vi "Active Power-Spectrum Method-v3_YCC.vi"() -> ()   [LabVIEW 2014]
uses:
  <vilib>/DAQmx/create/channels.llb/DAQmx Create Channel (AI-Voltage-Basic).vi
  <vilib>/DAQmx/configure/timing.llb/DAQmx Timing (Sample Clock).vi
  <vilib>/DAQmx/read.llb/DAQmx Read (Analog 1D DBL 1Chan NSamp).vi
panel:
  in  "Who's Data":enum16{"YCC", "PYW", "LCH", "YYH"}(ring)
  out "All Bead Response (V)":dbl[](array[numeric])
  out "Freq. Cut for fitting":dbl[](array[numeric])
  out "best fit PSD for Thermal background":dbl[](array[numeric])
  in  "Save?":bool
  in  "Volumn of glycerol":dbl
  in  "Volumn of water":dbl=1.0
  out "A scaling":dbl
  out "True Amplitude, A (nm)":dbl
  out "Sample size per cycle":dbl
  out "size(s)":i32
  out "SinePosition (um)":dbl[](array[numeric])
  out "ms to wait (ms)":dbl
  out "df (Hz)":dbl
  in  "time per cycle (s)":dbl=0.125
  in  "Fs,#points":dbl=800.0
  in  "Custum Fs (Hz)":i32
  in  "Sampling Rate (Hz)":T1(ring)=enum."131072"
  out "Axis":i32
  out "Real Current Commanded position (um)":dbl format="%0.5f"
  out "Sample size for all":dbl
  out "physical channels":tag
  out "stiffness from diffusion coeff.(pN/nm)":dbl
  in  "Temp (C)":dbl=25.0
  out "stiffness from friction coeff.(pN/nm)":dbl format="%#_6f"
  out "Diffusion coefficient, D (V^2/s)":dbl
  out "a1":dbl
  in  "bead height (um)":dbl=1.0
  in  "bead radius (um)":dbl=0.515
  out "Beta (V/um)":dbl
  out "fResponse (Hz)":dbl
  out "Wex":dbl
  out "Wth":dbl
  out "fc":dbl
  out "best fit parameters\n(XX,fc)":dbl[](array[numeric])
  in  "Freq End Cut":dbl=60000.0
  in  "Freq Strat Cut":dbl=50.0
  out "Frequency (Hz)\n0,df, 2df,...(n/2-1)Fs":dbl[](array[numeric])
  out "Avg. PSD":dbl[](array[numeric])
  out "Avg. completed":i32
  in  "Tab Control":enum32{"Page 1", "Time domain", "PSD"}(tab)
  out "XY Graph":T2(graph)
  out "XY Graph 3":cluster{"Time (s)":dbl[], "Position (um)":dbl[]}(graph)
  out "Bead Response Waveform":dbl[](graph)
  out "XY Graph 2":T3(graph)
  in  "Cycles to average":i32=64
  out "Sampling Rate (Hz)":i32=32000
  out "Need time (s)":dbl format="%.5f"
  in  "Amplitude, A (nm)":dbl=1000.0
  in  "f_drive (Hz)":dbl=32.0
  in  "Axis (Enum)":enum16{"x", "y", "z"}(ring)
  # "fcut=80k\nfs=131072"
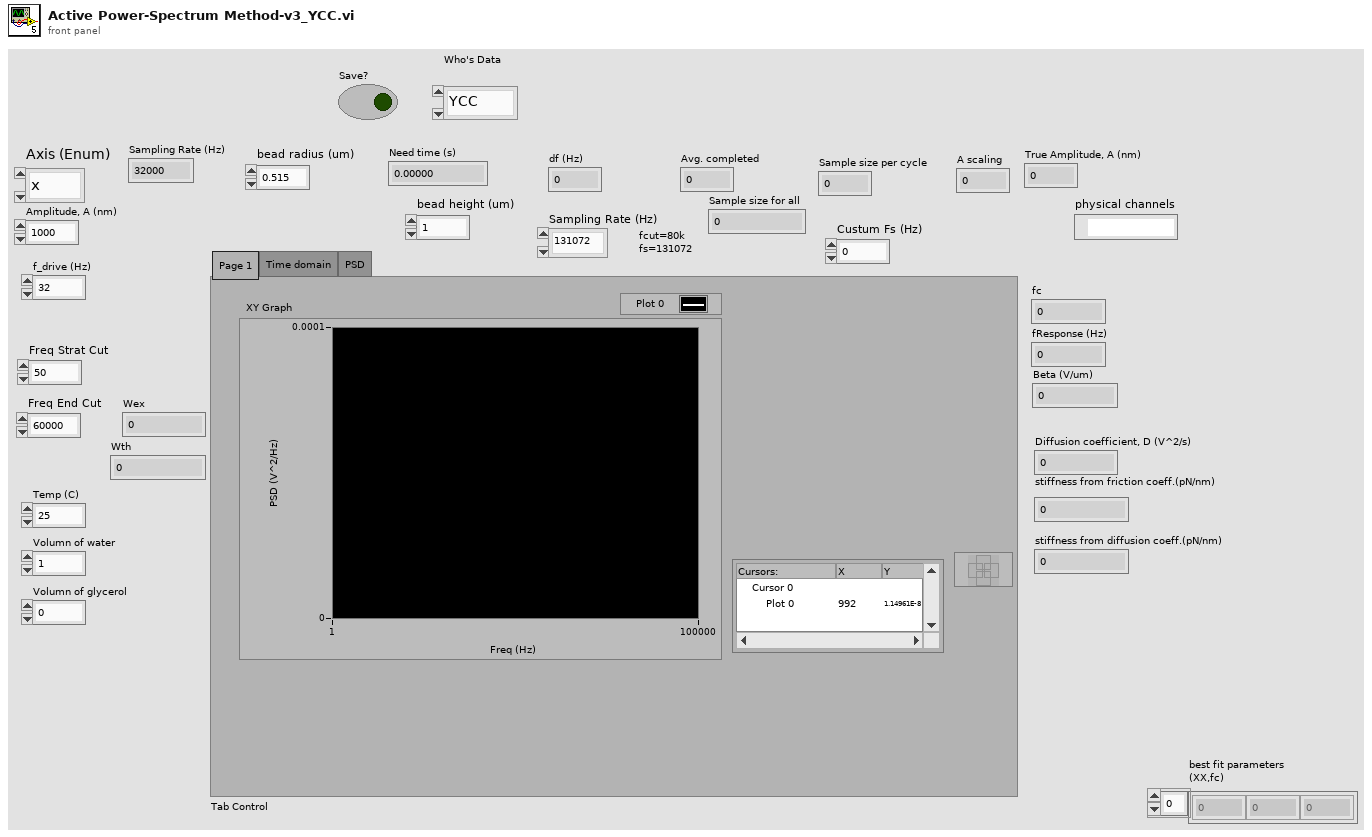
[diagram p1: front panel]
types:
  T1 = enum16{"custum", "16384", "32768", "65536", "131072", "262144"}
  T2 = cluster{"Frequency (Hz)\n0,df, 2df,...(n/2-1)Fs":dbl[], dbl[]}
  T3 = cluster{"Frequency (Hz)\n0,df, 2df,...(n/2-1)Fs":dbl[], dbl[]}[]
  T4 = cluster{"Time Array (s)":dbl[], "Position Array (um)":dbl[]}
  T5 = cluster{"Freq Cut":dbl[], "best nonlinear fit PSD":dbl[]}
  T6 = cluster{"Frequency (Hz)\n0,df, 2df,...(n/2-1)Fs":dbl[], "best nonlinear fit PSD":dbl[]}[]
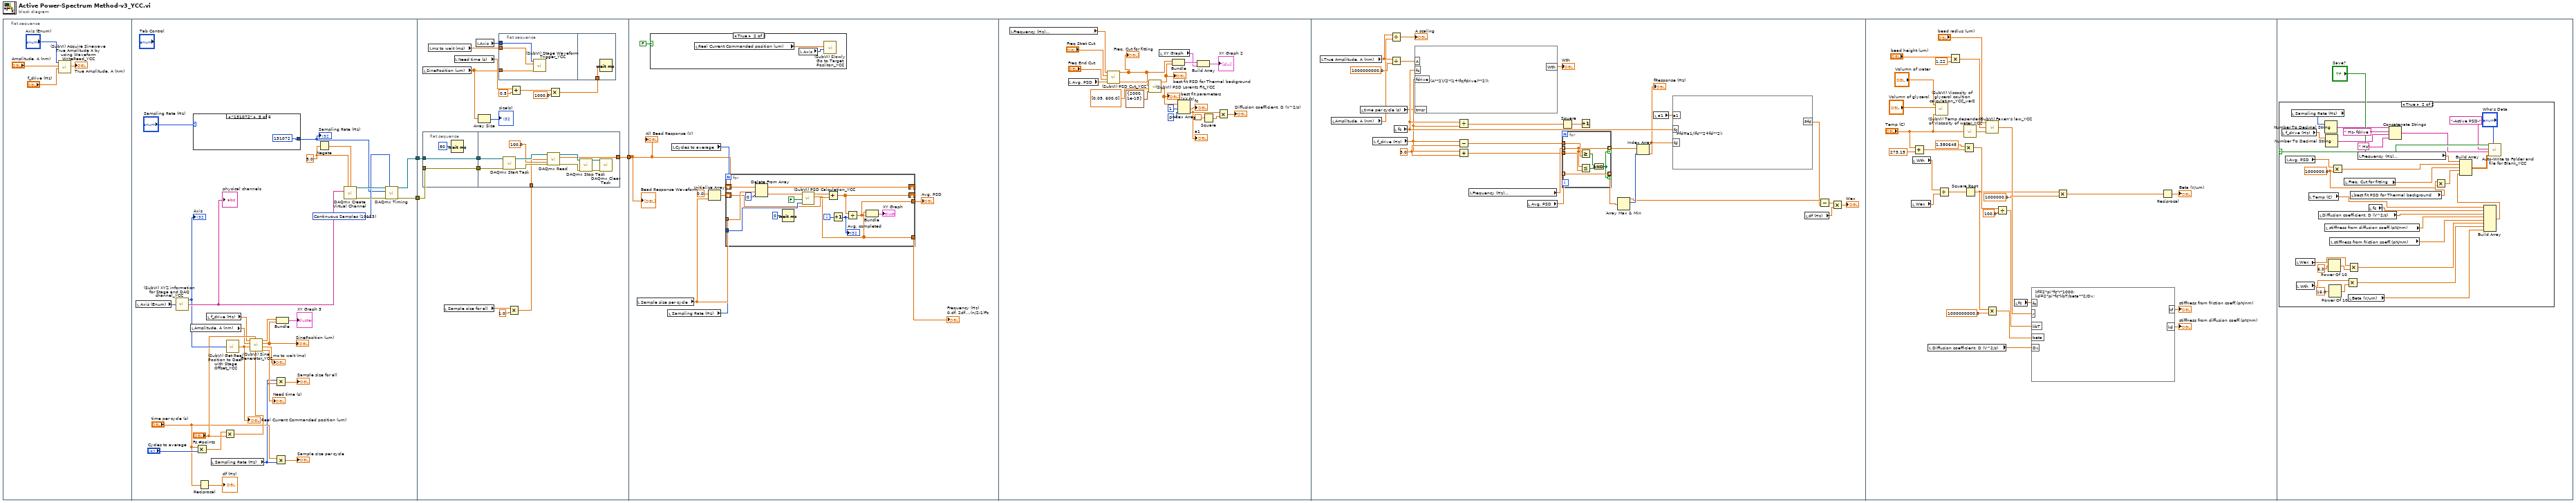
[diagram p0: block diagram]
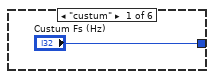
[diagram p2: hidden frame]
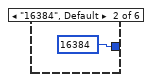
[diagram p3: hidden frame]
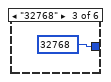
[diagram p4: hidden frame]
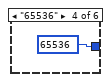
[diagram p5: hidden frame]
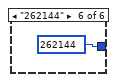
[diagram p6: hidden frame]
diagram:
  n1 = flat-sequence {
    tunnel: [w19] -> w3
    tunnel: [w18] -> w2
    tunnel: w3 -> [w59]
    tunnel: w2 -> [w58]
    tunnel: [w52] -> w1
    tunnel: w1 -> [w84]
    frame #0 {
      n2 = call "(SubVI) Acquire Sinewave True Amplitude A by using Waveform WriteRead_YCC.vi"("f_drive (Hz)"="f_drive (Hz)", "Amplitude, A (nm)"="Amplitude, A (nm)", "Axis  (Enum)"="Axis (Enum)") -> ("True Amplitude, A (nm)"=→"True Amplitude, A (nm)":dbl)  [unwired: 3 in, 1 out]
    }
    frame #1 {
      w31 = 10123 items=["Finite Samples"=10178, "Continuous Samples"=10123, "Hardware Timed Single Point"=12522] ("sample mode")
      w35 = 5.0 ("maximum value")
      n3 = local read "Axis (Enum)"() -> (w10:enum16{"x", "y", "z"})
      n4 = call "(SubVI) XYZ information for Stage and DAQ channel_YCC.vi"("Axis  (Enum)"=w10) -> ("physical channels"=w36:tag, "Axis"=w30:i32)  [unwired: 3 in]
      "physical channels" <- w36
      "Axis" <- w30
      n5 = local read "Amplitude, A (nm)"() -> (w9:dbl)
      n6 = case shown="\"131072\"" "Sampling Rate (Hz)" {
        tunnel: ["Custum Fs (Hz)" 16384 32768 65536 131072 262144] -> w27
        frame "custum" {
        }
        frame "16384", Default {
        }
        frame "32768" {
        }
        frame "65536" {
        }
        frame "131072" {
        }
        frame "262144" {
        }
      }
      "Sampling Rate (Hz)" <- w27
      n7 = Multiply(x="time per cycle (s)", y="Cycles to average") -> (x*y=w21:dbl)
      n8 = Reciprocal(x="time per cycle (s)") -> (1/x=→"df (Hz)":dbl)
      n9 = local read "f_drive (Hz)"() -> (w8:dbl)
      n10 = local read "Sampling Rate (Hz)"() -> (w15:i32)
      n11 = Multiply(x=w21, y="Fs,#points") -> (x*y=w20:dbl)
      n12 = call "(SubVI) Get Real Position to Deal with Stage Offset_YCC.vi"("Axis"=w30) -> ("Real Current Commanded position (um)"=w29:dbl)  [unwired: 3 in, 1 out]
      "Real Current Commanded position (um)" <- w29
      n13 = call "(SubVI) Sine Generator_YCC.vi"("Points to be generated"=w20, "fs (Hz)"="Fs,#points", "initial position (um)"=w29, "Amplitude, A (nm)"=w9, "f_drive (Hz)"=w8) -> ("Total Need time (s)"=w25:dbl, "waiting time (to write) (ms)"=→"ms to wait (ms)":dbl, "Position Array (um)"=w12:dbl[], "Time Array (s)"=w13:dbl[])  [unwired: 1 in]
      "Need time (s)" <- w25
      "SinePosition (um)" <- w12
      n14 = Multiply(x=w15, y=w25) -> (x*y=→"Sample size for all":dbl)
      n15 = Multiply(x="time per cycle (s)", y=w15) -> (x*y=→"Sample size per cycle":dbl)
      n16 = Bundle("Time Array (s)"=w13, "Position Array (um)"=w12) -> (→"XY Graph 3":T4)  [unwired: 1 in]
      n17 = Negate(x=w35) -> (-x=w34:dbl)
      n18 = call-poly <vilib>:"DAQmx Create Virtual Channel.vi"("maximum value"=w35, "minimum value"=w34, "physical channels"=w36) -> ("task out"=w33:refnum<k21>, "error out"=w32:errorcluster)  [unwired: 11 in]
      n19 = call-poly <vilib>:"DAQmx Timing.vi"("task/channels in"=w33, "sample mode"=w31, "rate"=w27, "error in"=w32) -> ("task out"=w19:refnum<k21>, "error out"=w18:errorcluster)  [unwired: 3 in, 7 out]
    }
    frame #2 {
      n20 = local read "SinePosition (um)"() -> (w43:dbl[])
      n21 = flat-sequence {
        tunnel: w58 -> [w61]
        tunnel: w59 -> [w62]
        tunnel: [w62] -> w48
        tunnel: [w61] -> w47
        tunnel: [w64] -> w52
        tunnel: w49 -> [w63]
        tunnel: w48 -> [w66]
        tunnel: w47 -> [w65]
        frame #0 {
          n22 = Wait (ms)(milliseconds to wait=u32 80) -> ()  [unwired: 1 out]
        }
        frame #1 {
          n23 = call <vilib>:"DAQmx Start Task.vi"("task/channels in"=w66, "error in"=w65) -> ("task out"=w72:refnum<k21>, "error out"=w73:errorcluster)  [unwired: 12 out]
          n24 = call-poly <vilib>:"DAQmx Read.vi"("task/channels in"=w72, "number of samples per channel"=w63, "timeout"=100.0, "error in"=w73) -> ("task out"=w69:refnum<k21>, "data"=w64:dbl[], "error out"=w71:errorcluster)  [unwired: 9 in]
          n25 = call <vilib>:"DAQmx Stop Task.vi"("task/channels in"=w69, "error in"=w71) -> ("task out"=w67:refnum<k21>, "error out"=w68:errorcluster)  [unwired: 12 in]
          n26 = call <vilib>:"DAQmx Clear Task.vi"("task in"=w67, "error in"=w68) -> ()  [unwired: 13 in, 1 out]
        }
      }
      n27 = local read "ms to wait (ms)"() -> (w57:dbl)
      n28 = local read "Sample size for all"() -> (w51:dbl)
      n29 = local read "Need time (s)"() -> (w46:dbl)
      n30 = local read "Axis"() -> (w56:i32)
      n31 = Array Size(array=w43) -> (size(s)=→"size(s)":i32)
      n32 = flat-sequence {
        tunnel: w57 -> [w76]
        tunnel: w56 -> [w75]
        tunnel: w43 -> [w74]
        tunnel: w54 -> [w77]
        frame #0 {
          n33 = call "(SubVI) Stage Waveform Trigger_YCC.vi"("Position Array (um)"=w74, "milliseconds to wait"=w76, "axis"=w75) -> ()  [unwired: 5 in]
        }
        frame #1 {
          n34 = Wait (ms)(milliseconds to wait=w77) -> ()  [unwired: 1 out]
        }
      }
      n35 = Multiply(x=w51, y=1.0) -> (x*y=w49:dbl)
      n36 = Add(x=w46, y=0.5) -> (x+y=w44:dbl)
      n37 = Multiply(x=w44, y=1000.0) -> (x*y=w54:dbl)
    }
    frame #3 {
      n38 = local read "Sample size per cycle"() -> (w83:dbl)
      n39 = case shown="True" FALSE {
        frame False {
        }
        frame True {
          n40 = local read "Real Current Commanded position (um)"() -> (w88:dbl)
          n41 = local read "Axis"() -> (w87:i32)
          n42 = call "(SubVI) Slowly Go to Target Posiiton_YCC.vi"("axis"=w87, "Target position (um)"=w88) -> ()  [unwired: 2 in, 4 out]
        }
      }
      n43 = local read "Sampling Rate (Hz)"() -> (w81:i32)
      n44 = local read "Cycles to average"() -> (w85:i32)
      n45 = Initialize Array(0.0 ("element"), w83) -> (w82:dbl[])
      n46 = for {
        N: w85 -> [_]
        shift-right: [w98] -> _
        shift-left: w84 -> [w101]
        tunnel: w83 -> [w100]
        shift-right: [w93] -> _
        shift-left: w82 -> [w95]
        tunnel: w81 -> [w96]
        tunnel: [w91] -> w80
        tunnel: [w90] -> w79
        i -> [w94]
        n47 = Delete From Array(array=w101, length=w100, index=0) -> (deleted portion=w97:dbl[], array with subset deleted=w98:dbl[])
        n48 = Wait (ms)(milliseconds to wait=u32 0) -> ()  [unwired: 1 out]
        n49 = call "(SubVI) PSD Calculation_YCC.vi"("sampling frequency (Hz)"=w96, "T=NI made PSD\nF=YCC made PSD"=FALSE ("T=NI made PSD\nF=YCC made PSD"), "QPD data"=w97) -> ("Frequency (Hz)\n0,df, 2df,...(n/2-1)Fs"=w91:dbl[], "Power Spectrum (V^2 rms) (V^2/Hz)"=w102:dbl[])  [unwired: 3 in]
        n50 = Add(x=w102, y=w95) -> (x+y=w93:dbl[])
        n51 = Increment(x=w94) -> (x+1=w92:i32)
        "Avg. completed" <- w92
        n52 = Divide(x=w93, y=w92) -> (x/y=w90:dbl[])
        n53 = Bundle("Frequency (Hz)\n0,df, 2df,...(n/2-1)Fs"=w91, w90) -> (→"XY Graph":T2)  [unwired: 1 in]
      }
      "Frequency (Hz)\n0,df, 2df,...(n/2-1)Fs" <- w80
      "Avg. PSD" <- w79
      "Bead Response Waveform" <- w84
      "All Bead Response (V)" <- w84
    }
    frame #4 {
      n54 = local read "Frequency (Hz)\n0,df, 2df,...(n/2-1)Fs"() -> (w108:dbl[])
      n55 = local read "Avg. PSD"() -> (w107:dbl[])
      n56 = call "(SubVI) PSD Cut_YCC.vi"("PSD"=w107, "Freq End Cut"="Freq End Cut", "Freq Strat Cut"="Freq Strat Cut", "Frequency (Hz)"=w108) -> ("PSD Cut"=w122:dbl[], "Freq Cut"=w105:dbl[])  [unwired: 2 in]
      "Freq. Cut for fitting" <- w105
      n57 = call "(SubVI) PSD Lorentz Fit_YCC.vi"("termination"=cluster{"max iteration":i32, "tolerance":dbl} {"max iteration"=2000, "tolerance"=1e-15}, "initial parameters"=dbl[] [0.05, 600.0], "Frequency (Hz)"=w105, "PSD (Vrms^2)"=w122) -> ("best fit parameters"=w116:dbl[], "best nonlinear fit PSD"=w119:dbl[])  [unwired: 2 in]
      "best fit parameters\n(XX,fc)" <- w116
      "best fit PSD for Thermal background" <- w119
      n58 = local read "XY Graph"() -> (w117:T2)
      n59 = Bundle("Freq Cut"=w105, "best nonlinear fit PSD"=w119) -> (w118:T5)  [unwired: 1 in]
      n60 = Index Array(array=w116, index #1=1 ("index"), index #2=0 ("index")) -> (element #1=→"fc":dbl, element #2=w110:dbl)
      "a1" <- w110
      n61 = Build Array(w118, w117) -> (→"XY Graph 2":T6)
      n62 = Square(x=3.141592653589793) -> (x^2=w111:dbl)
      n63 = Multiply(x=w110, y=w111) -> (x*y=→"Diffusion coefficient, D (V^2/s)":dbl)
    }
    frame #5 {
      w148 = 3.0 ("y")
      n64 = local read "True Amplitude, A (nm)"() -> (w127:dbl)
      n65 = local read "Amplitude, A (nm)"() -> (w126:dbl)
      n66 = local read "time per cycle (s)"() -> (w130:dbl)
      n67 = local read "f_drive (Hz)"() -> (w134:dbl)
      n68 = Divide(x=w127, y=w126) -> (x/y=→"A scaling":dbl)
      n69 = Divide(x=w127, y=1000000000.0) -> (x/y=w136:dbl)
      n70 = local read "fc"() -> (w135:dbl)
      n71 = formula code="Wth=(A**2)/(2*(1+(fc/fdrive)**2));"("A"=w136, "fc"=w135, "fdrive"=w134, "tmsr"=w130) -> ("Wth"=→"Wth":dbl)
      n72 = Divide(x=w135, y=w134) -> (x/y=w133:dbl)
      n73 = Subtract(x=w134, y=w148) -> (x-y=w147:dbl)
      n74 = Add(x=w134, y=w148) -> (x+y=w146:dbl)
      n75 = local read "Frequency (Hz)\n0,df, 2df,...(n/2-1)Fs"() -> (w149:dbl[])
      n76 = local read "Avg. PSD"() -> (w150:dbl[])
      n77 = Square(x=w133) -> (x^2=w132:dbl)
      n78 = for {
        tunnel: [w157] -> w145 mode=indexing if=w151
        tunnel: w150 -> [w157] mode=indexing
        tunnel: [w155] -> w144 mode=indexing if=w151
        tunnel: w149 -> [w155] mode=indexing
        tunnel: w147 -> [w156]
        tunnel: w146 -> [w154]
        n79 = Greater Or Equal?(x=w155, y=w156) -> (x >= y?=w153:bool)
        n80 = Less Or Equal?(x=w155, y=w154) -> (x <= y?=w152:bool)
        n81 = And(x=w153, y=w152) -> (x .and. y?=w151:bool)
      }
      n82 = Increment(x=w132) -> ()  [unwired: 1 out]
      n83 = Array Max & Min(array=w145) -> (max value=w141:dbl, max index (indices)=w143:i32)  [unwired: 2 out]
      n84 = Index Array(array=w144, index=w143) -> (element=w128:dbl)
      "fResponse (Hz)" <- w128
      n85 = local read "a1"() -> (w142:dbl)
      n86 = formula code="Pfd=a1/(fc**2+fd**2);"("a1"=w142, "fc"=w135, "fd"=w128) -> ("Pfd"=w129:dbl)
      n87 = local read "df (Hz)"() -> (w139:dbl)
      n88 = Subtract(x=w141, y=w129) -> (x-y=w140:dbl)
      n89 = Multiply(x=w140, y=w139) -> (x*y=→"Wex":dbl)
    }
    frame #6 {
      n90 = local read "Wex"() -> (w184:dbl)
      n91 = local read "Wth"() -> (w185:dbl)
      n92 = Add(x="Temp (C)", y=273.15) -> (x+y=w178:dbl)
      n93 = local read "Diffusion coefficient, D (V^2/s)"() -> (w171:dbl)
      n94 = call "(SubVI) Viscosity of glycerol soultion calculation_YCC_ver2.vi"("Volumn of water"="Volumn of water", "Volumn of glycerol"="Volumn of glycerol", "Temperature (C)"="Temp (C)") -> ()  [unwired: 4 in, 2 out]
      n95 = Divide(x=w185, y=w184) -> (x/y=w168:dbl)
      n96 = Multiply(x="bead height (um)", y=1.22) -> (x*y=w161:dbl)
      n97 = Multiply(x=1.380648, y=w178) -> (x*y=w177:dbl)
      n98 = call "(SubVI) Temp dependent of Viscosity of water_YCC.vi"("Temperature (C)"="Temp (C)") -> ("Viscosity (mPa*s)"=w164:dbl)  [unwired: 4 in]
      n99 = Square Root(x=w168) -> (sqrt(x)=w167:dbl)
      n100 = call "(SubVI) Faxen's law_YCC.vi"("viscosity (cP)"=w164, "bead height (um)"=w161, "bead radius (um)"="bead radius (um)") -> ("Faxen's law of friction coefficient (N/(m/s))"=w173:dbl)  [unwired: 2 in]
      n101 = Multiply(x=w167, y=1000000000.0) -> (x*y=w165:dbl)
      n102 = Divide(x=w177, y=100.0) -> (x/y=w175:dbl)
      n103 = local read "fc"() -> (w174:dbl)
      n104 = formula code="kf=2*pi*fc*r*1000;\nkd=2*pi*fc*kbT/beta**2/Dv;"("fc"=w174, "r"=w173, "kbT"=w175, "beta"=w165, "Dv"=w171) -> ("kf"=→"stiffness from friction coeff.(pN/nm)":dbl, "kd"=→"stiffness from diffusion coeff.(pN/nm)":dbl)
      n105 = Multiply(x=w167, y=1000000.0) -> (x*y=w172:dbl)
      n106 = Reciprocal(x=w172) -> (1/x=→"Beta (V/um)":dbl)
    }
    frame #7 {
      n107 = case shown="True" "Save?" {
        selector: "Save?" -> [_ w219]
        frame False {
        }
        frame True {
          w197 = 1000000.0 ("y")
          n108 = local read "f_drive (Hz)"() -> (w204:dbl)
          n109 = local read "Avg. PSD"() -> (w200:dbl[])
          n110 = local read "Sampling Rate (Hz)"() -> (w207:i32)
          n111 = local read "Wex"() -> (w190:dbl)
          n112 = local read "Wth"() -> (w188:dbl)
          n113 = local read "Temp (C)"() -> (w208:dbl)
          n114 = local read "Diffusion coefficient, D (V^2/s)"() -> (w214:dbl)
          n115 = Number To Decimal String(number=w207) -> (decimal integer string=w206:string)  [unwired: 1 in]
          n116 = local read "stiffness from diffusion coeff.(pN/nm)"() -> (w213:dbl)
          n117 = Number To Decimal String(number=w204) -> (decimal integer string=w203:string)  [unwired: 1 in]
          n118 = Power Of 10(x=6.0) -> (10^x=w191:dbl)
          n119 = Power Of 10(x=16.0) -> (10^x=w194:dbl)
          n120 = local read "stiffness from friction coeff.(pN/nm)"() -> (w212:dbl)
          n121 = Multiply(x=w200, y=w197) -> (x*y=w199:dbl[])
          n122 = local read "Freq. Cut for fitting"() -> (w216:dbl[])
          n123 = Multiply(x=w188, y=w194) -> (x*y=w187:dbl)
          n124 = Multiply(x=w190, y=w191) -> (x*y=w189:dbl)
          n125 = local read "Beta (V/um)"() -> (w195:dbl)
          n126 = local read "best fit PSD for Thermal background"() -> (w198:dbl[])
          n127 = local read "Frequency (Hz)\n0,df, 2df,...(n/2-1)Fs"() -> (w217:dbl[])
          n128 = local read "fc"() -> (w215:dbl)
          n129 = Concatenate Strings(w206, " Hz- fdrive " ("string"), w203, " Hz" ("string")) -> (w201:string)
          n130 = Multiply(x=w198, y=w197) -> (x*y=w196:dbl[])
          n131 = Build Array(w208, w215, w214, w213, w212, w189, w187, w195) -> (w211:dbl[])
          n132 = Build Array(w217, w199, w216, w196, w211) -> (w210:dbl[][])
          n133 = call "Auto-Write to Folder and file for Blank_YCC.vi"("Who's Data"="Who's Data", "data to be saved"=w210, "File name add to the end \n(height)"=w201, "Title"="-Active PSD-", "Save?"=w219) -> ()  [unwired: 3 in, 2 out]
        }
      }
    }
  }
